vi "NavigationDefensive.vi"(8 "error in (no error)":errorcluster, 11 "Game in":refnum<class "Game.lvclass">) -> (0 "error out":errorcluster, 3 "Game out":refnum<class "Game.lvclass">)   [LabVIEW 2020, in "Game.lvclass"]
uses:
  Game.lvclass
  Parameters_class/Parameters.lvclass
  Ally_class/Ally.lvclass
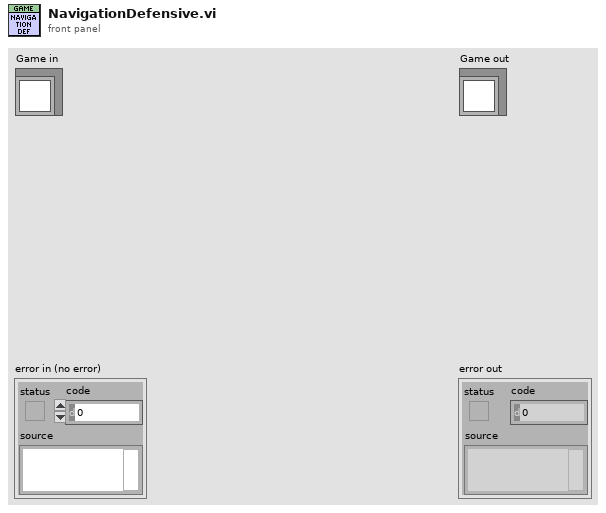
[diagram p1: front panel]
types:
  T1 = typedef "AI Input.ctl" = cluster{"our_robots":T2[], "enemy_robots":T2[], "balls":T9[], "geometry":T10, "IA Judge":T11, "Received Timestamp":timestamp, "Events":T13}
  T2 = typedef "AI Robot.ctl" = cluster{"id":u32, "function":T3, "x":dbl, "y":dbl, "orientation":dbl, "v_tangent":dbl, "v_normal":dbl, "v_ang":dbl, "kick_x":dbl, "kick_z":dbl, "dribble":bool, "Timestamp":timestamp, "estimatives":T4, "dest_x_kick":dbl, "dest_y_kick":dbl, "Gap Coord":dbl[], "States":T5, "Path ":dbl[][], "Path  Smooth":dbl[][], "Dest":T6, "vx_desired":dbl, "vy_desired":dbl, "slowBehavior":bool, "VSSStates":T8}
  T3 = typedef "Functions Enum.ctl" = enum16{"2nd Striker", "Attacker", "Goalie", "Defender", "Striker", "Goto 0", "Dummy", "Kicker", "ZigZag 0", "ZigZag 1", "ZigZag 2", "ZigZag 3", "ZigZag 4", "ZigZag 5", "ZigZag 6", "ZigZag 7", "ZigZag 8", ""}
  T4 = typedef "estimatives.ctl" = cluster{"est_v_tangent":dbl, "est_v_normal":dbl, "est_vx":dbl, "est_vy":dbl, "Pos Robot Est":dbl[], "est_v_ang":dbl}
  T5 = typedef "AttackerStates.ctl" = enum16{"Pass", "GoToTangent", "BallGetting", "GoToKick", ""}
  T6 = typedef "PathDests.ctl" = T7[]
  T7 = typedef "PathDest.ctl" = cluster{"dest_x":dbl, "dest_y":dbl, "dest_orientation":dbl, "dest_vel":dbl}
  T8 = typedef "VSSAttackerStates.ctl" = enum16{"Pass", "GoToTangent", "BallGetting", "GoToKick", "Rotate anti-clockwise", "Rotate Clockwise", ""}
  T9 = typedef "AI Ball.ctl" = cluster{"x":dbl, "y":dbl, "timestamp":timestamp, "Vel_x":dbl, "Vel_y":dbl, "Pos Bola Est":dbl[], "Valid":bool, "z":dbl, "Vel_z":dbl}
  T10 = typedef "Field Size.ctl" = cluster{"line_width":u32, "field_length":u32, "field_width":u32, "boundary_width":u32, "referee_width":u32, "goal_width":u32, "goal_depth":u32, "goal_wall_width":u32, "center_circle_radius":u32, "defense_radius":u32, "defense_stretch":u32, "free_kick_from_defense_dist":u32, "penalty_spot_from_field_line_dist":u32, "penalty_line_from_spot_dist":u32}
  T11 = typedef "AI Judge.ctl" = cluster{"stage":string, "command":string, "our_goalie_id":dbl, "enemy_goalie_id":dbl, "command enum":T12, "Time":enum16{"Azul", "Amarelo"}}
  T12 = typedef "Command Enum.ctl" = enum16{"Halt", "Stop", "Force Start", "PKA Normal Start", "Prepare Kickoff Ally", "PKE Normal Start", "Prepare Kickoff Enemy", "Prepare Penalty Ally", "PPA Normal Start", "Prepare Penalty Enemy", "PPE Normal Start", "Direct Free Enemy", "Direct Free Ally", "Indirect Free Enemy", "Indirect Free Ally", "Timeout Enemy", "Timeout Ally", "Goal Enemy", "Goal Ally", "Ball Placement Enemy", "Ball Placement Ally", "Normal Half Time", "Extra Time Break", "Extra Half Time", "None", "Post Game"}
  T13 = typedef "Events.ctl" = cluster{"Touch":bool, "Ball out":bool, "id touch":dbl, "Ball out of \nVision":bool, "Ball inside \nGoalie area":bool, "Robot not responding":bool, "Robots responding status":dbl[], "Enemy Ball \nPossession":bool, "Pass State":bool, "id end of pass":dbl, "Kick":bool, "Id ini Possession":dbl, "Ball Possesion":bool, "Id Possesion":dbl, "Direct Kick":bool, "2nd Strk Ativo":bool}
  T14 = cluster{"(Kc)":dbl, "(Ti, min)":dbl, "(Td, min)":dbl}
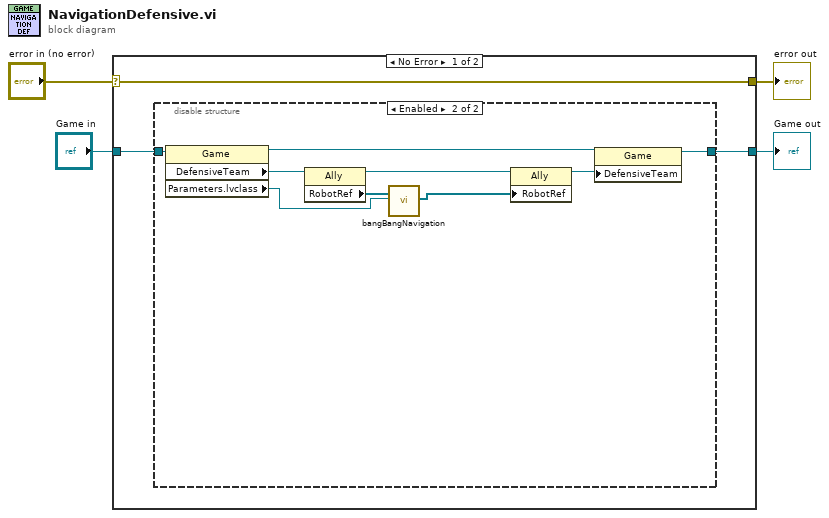
[diagram p0: block diagram]
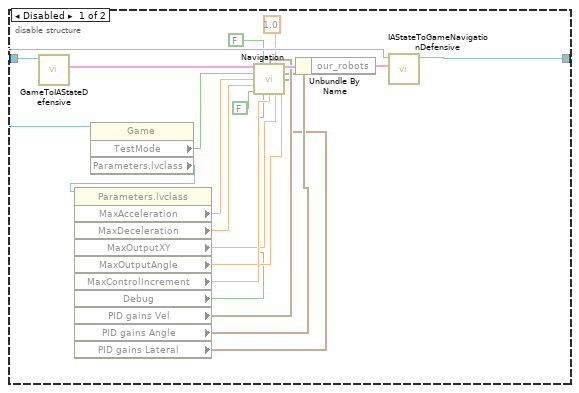
[diagram p2: hidden frame]
diagram:
  n1 = case shown="No Error" "error in (no error)" {
    selector: "error in (no error)" -> [w7 w37]
    tunnel: [w7 w37] -> w3
    tunnel: [w6 w36] -> w1
    tunnel: "Game in" -> [w5 w36]
    frame No Error {
      n2 = disable-structure shown="Enabled" {
        disable-tunnel: [w24 w29] -> w6
        disable-tunnel: w5 -> [w22 w35]
        frame Disabled {
          n3 = call "GameToIAStateDefensive.vi"("Game in"=w22) -> ("IA State out"=w23:T1)  [unwired: 8 in, 2 out]
          n4 = property class="Game"(reference=w22) -> ("TestMode"=w12:bool, "Parameters.lvclass"=w21:refnum<class "Parameters.lvclass">)  [unwired: 1 in, 2 out]
          n5 = property class="Parameters.lvclass"(reference=w21) -> ("MaxAcceleration"=w20:dbl, "MaxDeceleration"=w19:dbl, "MaxOutputXY"=w17:dbl, "MaxOutputAngle"=w16:dbl, "MaxControlIncrement"=w18:dbl, "Debug"=w14:bool, "PID gains Vel"=w13:T14, "PID gains Angle"=w9:cluster{"(Kc)":dbl, "(Ki)":dbl, "(Kd)":dbl}, "PID gains Lateral"=w8:cluster{"(Kc)":dbl, "(Ki)":dbl, "(Kd)":dbl})  [unwired: 1 in, 2 out]
          n6 = call "Navigation.vi"("IA State Output in"=w23, "Penalty Shoot Out?"=FALSE, "PID gains Vel"=w13, "VelNearBall"=1.0, "Test Mode"=w12, "PID gains Angle"=w9, "a1"=w20, "PID gains Lateral"=w8, "a3"=w19, "GoTo Navigation"=FALSE, "Debug"=w14, "output inc"=w18, "output xy"=w17, "output angle"=w16) -> ("IA State Output out"=w26:T1)  [unwired: 1 in]
          n7 = Unbundle By Name(w26) -> ("our_robots"=w25:T2[])
          n8 = call "IAStateToGameNavigationDefensive.vi"("our_robots"=w25, "Game in"=w22) -> ("Game out"=w24:refnum<class "Game.lvclass">)  [unwired: 8 in, 1 out]
        }
        frame Enabled {
          n9 = property class="Game"(reference=w35) -> (reference out=w28:refnum<class "Game.lvclass">, "DefensiveTeam"=w34:refnum<class "Ally.lvclass">, "Parameters.lvclass"=w32:refnum<class "Parameters.lvclass">)  [unwired: 1 in, 1 out]
          n10 = property class="Ally"(reference=w34) -> (reference out=w31:refnum<class "Ally.lvclass">, "RobotRef"=w33:refnum<class "Robot.lvclass">[])  [unwired: 1 in, 1 out]
          n11 = call "bangBangNavigation.vi"("RobotRef"=w33, "Parameters.lvclass"=w32) -> ("RoboRef"=w30:refnum<class "Robot.lvclass">[])  [unwired: 15 in, 2 out]
          n12 = property class="Ally"(reference=w31, "RobotRef"=w30) -> (reference out=w27:refnum<class "Ally.lvclass">)  [unwired: 1 in, 1 out]
          n13 = property class="Game"(reference=w28, "DefensiveTeam"=w27) -> (reference out=w29:refnum<class "Game.lvclass">)  [unwired: 1 in, 1 out]
        }
      }
    }
    frame Error {
    }
  }
  "error out" <- w3
  "Game out" <- w1
